vi "Check command.vi"(4 "error in (no error)":errorcluster, 5 "timeout in ms (-1)":i32=-1, 6 "Is connected":bool, 7 "Module mailbox":T1) -> (0 "error out":errorcluster, 1 "Command Data":variant, 2 "Command":T2)   [LabVIEW 2024, in "THz source modeule.lvlib"]
uses:
  THz source modeule.lvlib
  ctl/THz commands enum.ctl
  <userlib>/MatS Libs/MatS Mailman/TypeDefs/Mailbox ref.ctl
  ctl/THz Message for module.ctl
  <userlib>/MatS Libs/MatS Libs.lvlib
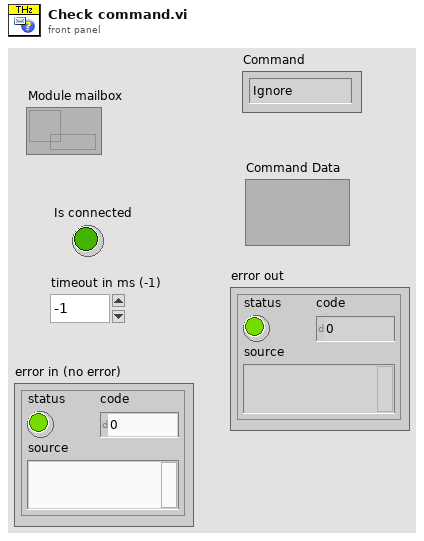
[diagram p1: front panel]
types:
  T1 = typedef "MatS Libs.lvlib/Mailbox ref.ctl" = refnum<queue>
  T2 = typedef "THz source modeule.lvlib/THz commands enum.ctl" = enum16{"Ignore", "Connect", "Update", "Set parameters", "Disconnect", "End"}
  T3 = typedef "THz source modeule.lvlib/THz Message for module.ctl" = cluster{"Command":T2, "Data":variant}
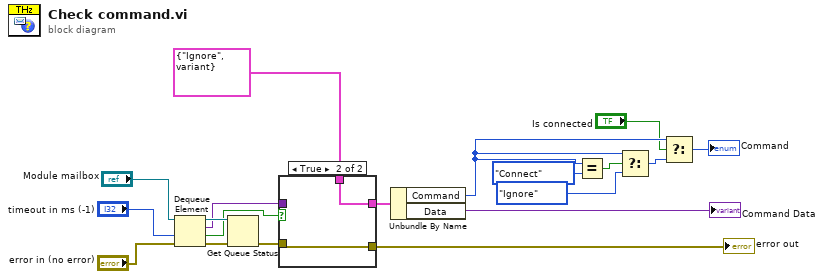
[diagram p0: block diagram]
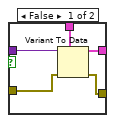
[diagram p2: hidden frame]
diagram:
  n1 = Dequeue Element(queue="Module mailbox", timeout in ms (-1)="timeout in ms (-1)", error in (no error)="error in (no error)") -> (queue out=w5:T1, element=w4:variant, timed out?=w1:bool, error out=w6:errorcluster)
  n2 = Get Queue Status(queue=w5, error in (no error)=w6) -> (error out=w3:errorcluster)  [unwired: 1 in, 7 out]
  n3 = case shown="True" w1 {
    tunnel: [w24 w25] -> w18
    tunnel: T3 {"Command"=enum."Ignore", "Data"=variant} ("Msg for THz module") -> [w23 w25]
    tunnel: w4 -> [w22 _]
    tunnel: w3 -> [w21 w26]
    tunnel: [w20 w26] -> w2
    frame False {
      n4 = Variant To Data(error in=w21, type=w23, Variant=w22) -> (data=w24:T3, error out=w20:errorcluster)
    }
    frame True {
    }
  }
  "error out" <- w2
  n5 = Unbundle By Name(w18) -> ("Command"=w14:T2, "Data"=→"Command Data":variant)
  n6 = Equal?(x=w14, y=THz_commands_enum."Connect" ("Command")) -> (x = y?=w15:bool)
  n7 = Select(t=w14, s=w15, f=THz_commands_enum."Ignore" ("Command")) -> (s? t:f=w16:T2)
  n8 = Select(t=w14, s="Is connected", f=w16) -> (s? t:f=→"Command":T2)
